vi "Shutdown HW.vi"(8 "error in (no error)":errorcluster, 11 "Sensor in":refnum<class "Sensor.lvclass">) -> (0 "error out":errorcluster, 3 "Sensor out":refnum<class "Sensor.lvclass">)   [LabVIEW 2020, in "Sensor.lvclass"]
uses:
  Sensor.lvclass
  General Hardware.lvclass
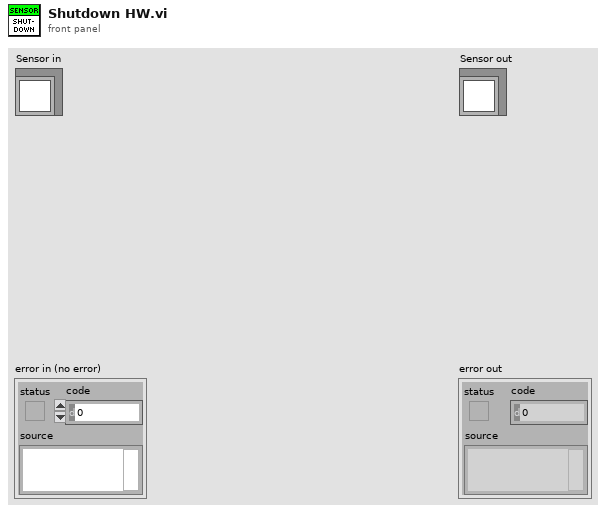
[diagram p1: front panel]
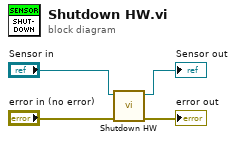
[diagram p0: block diagram]
diagram:
  n1 = call-parent "Shutdown HW.vi"("error in (no error)"="error in (no error)", "General Hardware in"="Sensor in") -> ("error out"=→"error out":errorcluster, "General Hardware out"=→"Sensor out":refnum<class "Sensor.lvclass">)  [unwired: 8 in]
